vi "Prompt for Step--UI Interlocks.vi"(8 "error in (no error)":errorcluster, 10 "Control Ref Map":map{string, refnum<vi>}(c390), 11 "Image Assertion in":refnum<class "Image Assertion.lvclass">) -> (0 "error out":errorcluster, 2 "Step Valid?":bool, 3 "Image Assertion out":refnum<class "Image Assertion.lvclass">)   [LabVIEW 2020, in "MacroAssert.lvlib" / "Image Assertion.lvclass"]
doc: "Enables or disables buttons within the \"Prompt for Step\" VI according to the current state of the system."
uses:
  Image Assertion.lvclass
  Image Assertion.lvclass/Image Assertion.ctl
  <userlib>/_MGI/Application Control/MGI Gray if/MGI Gray if False.vi
  MacroAssert.lvlib
  Image Assertion Type.ctl
  Support/Get Control Reference by Label (1D STR).vi
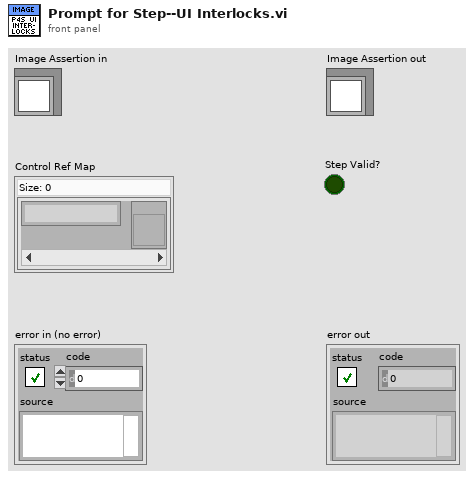
[diagram p1: front panel]
types:
  T1 = typedef "MacroAssert.lvlib/Image Assertion.lvclass/Image Assertion Type.ctl" = enum16{"Control Image", "VI Image", "Window Image", "Cursor Icon"}
  T2 = enum8{"Enabled", "Disabled", "Disabled and Grayed Out"}
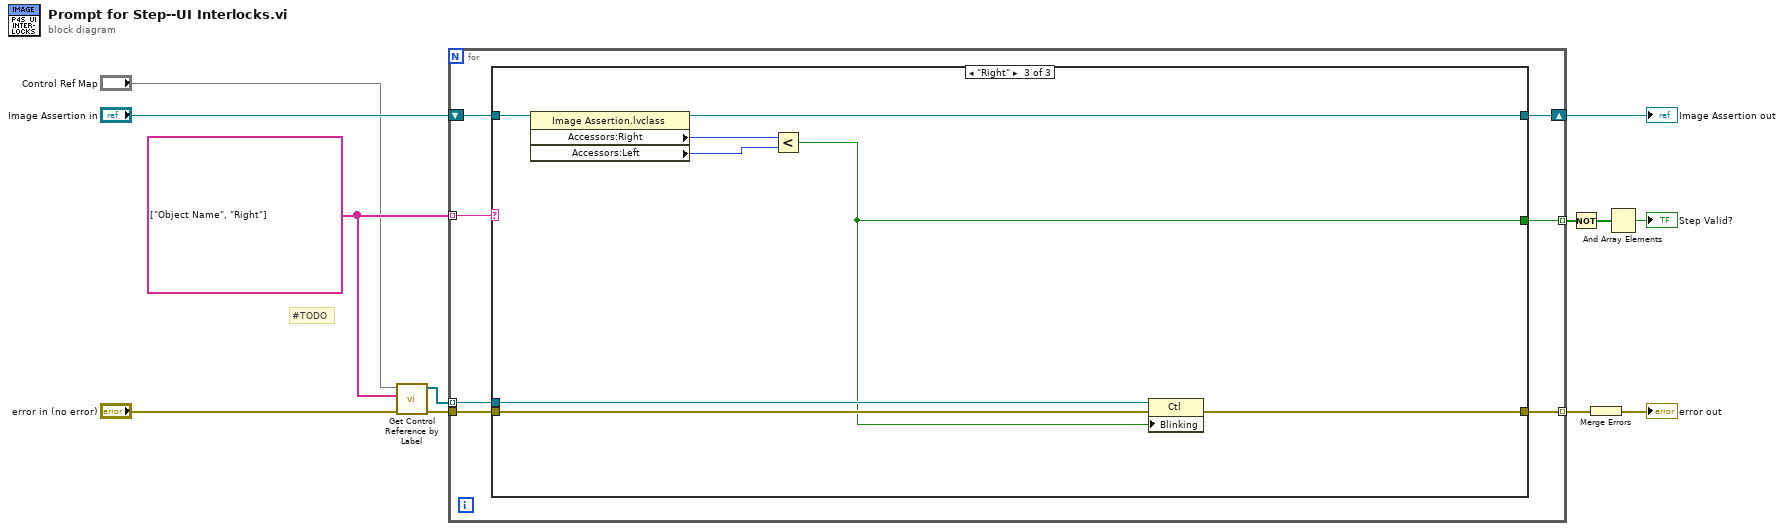
[diagram p0: block diagram]
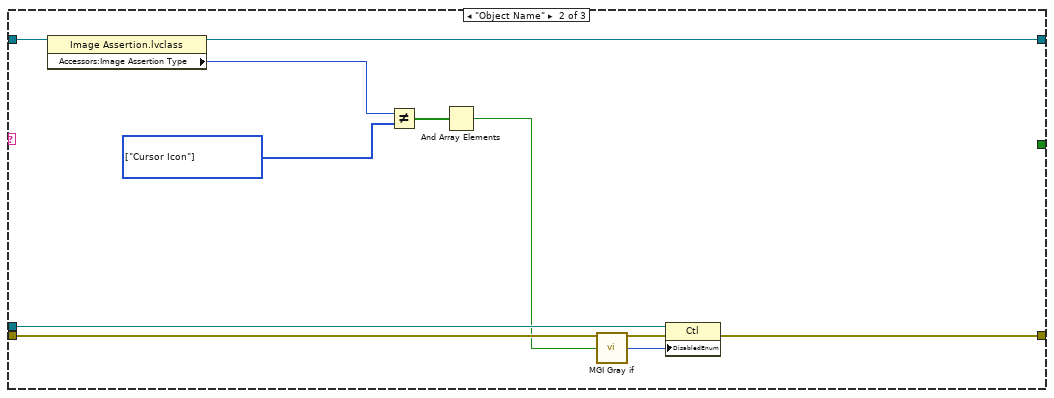
[diagram p3: hidden frame]
diagram:
  w11 = string[] ["Object Name", "Right"]
  # "#TODO"
  n1 = call-poly "Get Control Reference by Label.vi"("error in (no error)"="error in (no error)", "Control Names"=w11, "Control Ref Map"="Control Ref Map") -> ("error out"=w10:errorcluster, "Control Refs"=w9:refnum<vi>[])  [unwired: 6 in, 1 out]
  n2 = for {
    shift-right: [w16] -> w4
    shift-left: "Image Assertion in" -> [w19]
    tunnel: w11 -> [w18] mode=indexing
    tunnel: [w17] -> w12 mode=indexing
    tunnel: w10 -> [w15]
    tunnel: w9 -> [w14] mode=indexing
    tunnel: [w13] -> w3 mode=indexing
    n3 = case shown="\"Right\"" w18 {
      tunnel: w19 -> [w20 w31 w39]
      tunnel: w15 -> [w21 w29 w37]
      tunnel: [w21 w28 w36] -> w17
      tunnel: [w20 w30 w38] -> w16
      tunnel: w14 -> [_ w27 w35]
      tunnel: [_ _ w32] -> w13
      frame Default {
      }
      frame "Object Name" {
        w25 = T1[] [enum."Cursor Icon"] items=["Control Image", "VI Image", "Window Image", "Cursor Icon"]
        n4 = property class="Image Assertion.lvclass"(reference=w31) -> (reference out=w30:refnum<class "Image Assertion.lvclass">, "Accessors:Image Assertion Type"=w26:T1)  [unwired: 1 in, 1 out]
        n5 = Not Equal?(x=w26, y=w25) -> (x != y?=w24:bool[])
        n6 = And Array Elements(Boolean array=w24) -> (logical AND=w23:bool)
        n7 = call-poly <userlib>:"MGI Gray if.vi"("Boolean"=w23) -> ("Disabled"=w22:T2)
        n8 = property class="Ctl"(reference=w27, error in=w29, "DisabledEnum"=w22) -> (error out=w28:errorcluster)  [unwired: 1 out]
      }
      frame "Right" {
        n9 = property class="Image Assertion.lvclass"(reference=w39) -> (reference out=w38:refnum<class "Image Assertion.lvclass">, "Accessors:Right"=w34:i16, "Accessors:Left"=w33:i16)  [unwired: 1 in, 1 out]
        n10 = Less?(x=w34, y=w33) -> (x < y?=w32:bool)
        n11 = property class="Ctl"(reference=w35, error in=w37, "Blinking"=w32) -> (error out=w36:errorcluster)  [unwired: 1 out]
      }
    }
  }
  "Image Assertion out" <- w4
  n12 = Not(x=w3) -> (.not. x?=w2:bool[])
  n13 = Merge Errors(w12) -> (→"error out":errorcluster)
  n14 = And Array Elements(Boolean array=w2) -> (logical AND=→"Step Valid?":bool)
